vi "Parallel.vi"() -> ()   [LabVIEW 2023]
panel:
  out "Waveform Chart 2":dbl(graph)
  in  "Stop Button":bool
  out "Waveform Chart":dbl(graph)
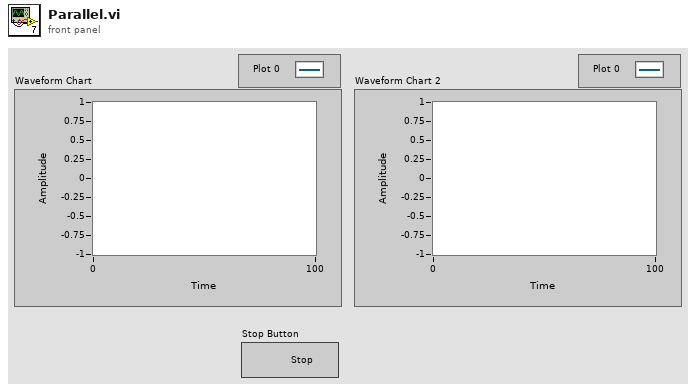
[diagram p1: front panel]
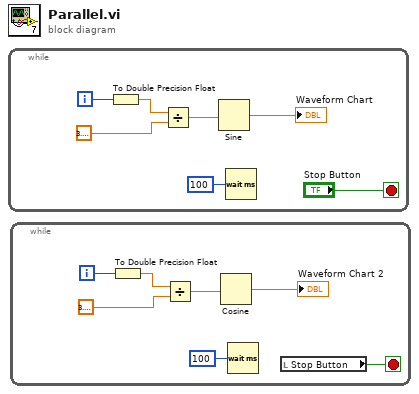
[diagram p0: block diagram]
diagram:
  n1 = while {
    i -> [w7]
    stop <- "Stop Button" stop-if-true
    n2 = To Double Precision Float(number=w7) -> (double precision float=w6:dbl)
    n3 = Divide(x=w6, y=3.141592653589793) -> (x/y=w2:dbl)
    n4 = Sine(x=w2) -> (sin(x)=→"Waveform Chart":dbl)
    n5 = Wait (ms)(milliseconds to wait=u32 100) -> ()  [unwired: 1 out]
  }
  n6 = while {
    i -> [w14]
    stop <- w8 stop-if-true
    n7 = To Double Precision Float(number=w14) -> (double precision float=w13:dbl)
    n8 = Divide(x=w13, y=3.141592653589793) -> (x/y=w10:dbl)
    n9 = Cosine(x=w10) -> (cos(x)=→"Waveform Chart 2":dbl)
    n10 = Wait (ms)(milliseconds to wait=u32 100) -> ()  [unwired: 1 out]
    n11 = local read "Stop Button"() -> (w8:bool)
  }
